vi "CPU_Load.vi"() -> (1 "System Resources:CPUs:Interrupt Load":u32[](array[numeric]), 2 "System Resources:CPUs:Total Load":u32[](array[numeric]), 3 "System Resources:CPUs:Count":i32, 5 "waveform cluster":T1)   [LabVIEW 2013]
uses:
  <vilib>/nisyscfg/Find Hardware.vi
  <resource>/objmgr/nisysapi.rc
  <vilib>/nisyscfg/nisyscfg.lvlib
panel:
  in  "Stop Button":bool
  out "Waveform Chart":cluster{dbl, dbl}(graph)
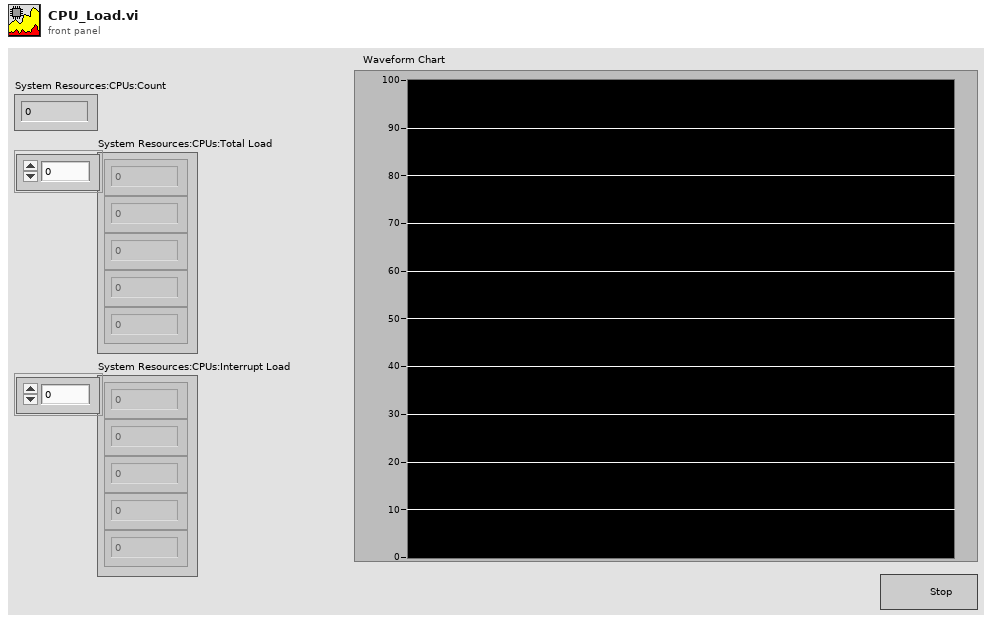
[diagram p1: front panel]
types:
  T1 = cluster{"Numeric Control":dbl, "Numeric Control":dbl}
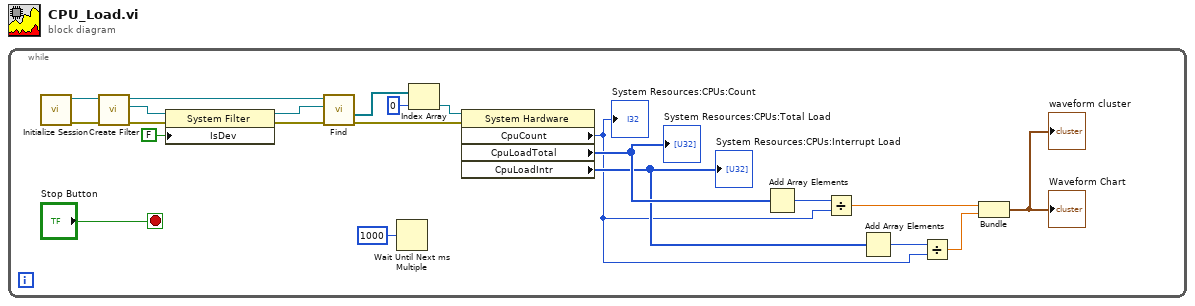
[diagram p0: block diagram]
diagram:
  n1 = while {
    stop <- "Stop Button" stop-if-true
    n2 = call <vilib>:"Initialize Session.vi"() -> ("error out"=w20:errorcluster, "Session out"=w21:refnum<k21>)  [unwired: 10 in]
    n3 = call <vilib>:"Create Filter.vi"("error in (no error)"=w20, "Session in"=w21) -> ("error out"=w22:errorcluster, "Filter out"=w18:refnum<k20>, "Session out"=w19:refnum<k21>)  [unwired: 7 in]
    n4 = property class="System Filter"(reference=w18, error in=w22, "IsDev"=FALSE ("Is Device")) -> (reference out=w17:refnum<k20>, error out=w16:errorcluster)
    n5 = call-poly <vilib>:"Find.vi"("error in (no error)"=w16, "Filter in"=w17, "Session in"=w19) -> ("error out"=w12:errorcluster, "Resources out"=w11:refnum<k20>[])  [unwired: 5 in, 2 out]
    n6 = Wait Until Next ms Multiple(millisecond multiple=u32 1000) -> ()  [unwired: 1 out]
    n7 = Index Array(array=w11, index=0) -> (element=w14:refnum<k20>)
    n8 = property class="System Hardware"(reference=w14, error in=w12) -> ("CpuCount"=w5:i32, "CpuLoadTotal"=w9:u32[], "CpuLoadIntr"=w6:u32[])  [unwired: 2 out]
    "System Resources:CPUs:Count" <- w5
    "System Resources:CPUs:Total Load" <- w9
    "System Resources:CPUs:Interrupt Load" <- w6
    n9 = Add Array Elements(numeric array=w9) -> (sum=w8:u32)
    n10 = Divide(x=w8, y=w5) -> (x/y=w4:dbl)
    n11 = Add Array Elements(numeric array=w6) -> (sum=w7:u32)
    n12 = Divide(x=w7, y=w5) -> (x/y=w3:dbl)
    n13 = Bundle(w4, w3) -> (→"Waveform Chart" →"waveform cluster":cluster{dbl, dbl})  [unwired: 1 in]
  }
